vi "FetchImageSet (SubVI).vi"(8 "error in (no error)":errorcluster, 10 "Naming Convention":string="*.png", 11 "Images Directory":path=path "E:/XYZstage+Camera_CollectedImages/12-16-2016/noStaveMount/toolingpins_images") -> (0 "error out":errorcluster, 2 "Image Array":T1[](array[typedef]), 3 "Filenames Array":string[](array[string]))   [LabVIEW 2016]
uses:
  <vilib>/vision/Image Controls.llb/IMAQ Image.ctl
  <vilib>/regexp/Match Regular Expression.xnode
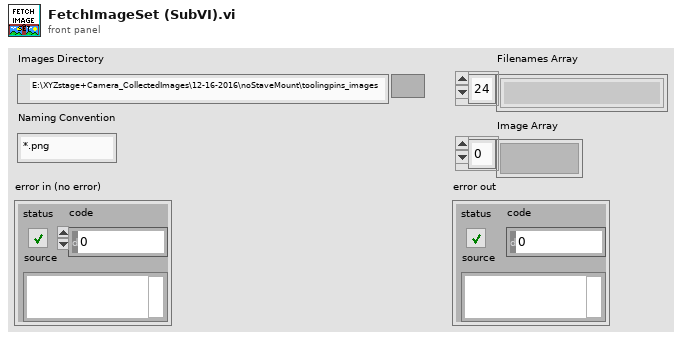
[diagram p1: front panel]
types:
  T1 = typedef "IMAQ Image.ctl" = refnum<image>
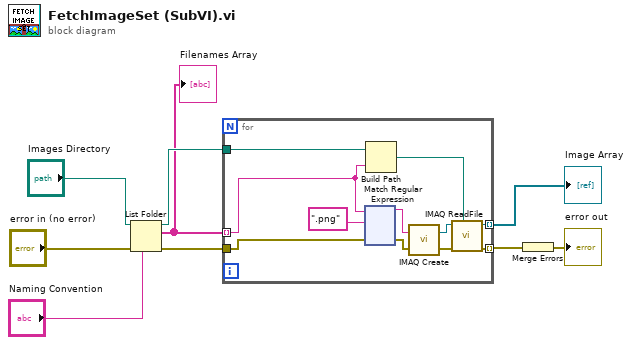
[diagram p0: block diagram]
diagram:
  n1 = List Folder(path="Images Directory", pattern="Naming Convention", error in="error in (no error)") -> (path out=w5:path, filenames=w1:string[], error out=w6:errorcluster)  [unwired: 1 in, 1 out]
  "Filenames Array" <- w1
  n2 = for {
    tunnel: w1 -> [w14] mode=indexing
    tunnel: w5 -> [w20]
    tunnel: w6 -> [w11]
    tunnel: [w16] -> w8 mode=indexing
    tunnel: [w15] -> w7 mode=indexing
    n3 = xnode "Match Regular Expression"("input string"=w14, "regular expression"=".png", "error in"=w11) -> ("before match"=w12:string, "error out"=w10:errorcluster)  [unwired: 3 in, 3 out]
    n4 = Build Path(base path=w20, name or relative path=w14) -> (appended path=w17:path)
    n5 = call "IMAQ Create"("Image Name"=w12, "error in (no error)"=w10) -> ("New Image"=w18:T1, "error out"=w19:errorcluster)  [unwired: 3 in]
    n6 = call "IMAQ ReadFile"("File Path"=w17, "error in (no error)"=w19, "Image"=w18) -> ("error out"=w15:errorcluster, "Image Out"=w16:T1)  [unwired: 4 in, 3 out]
  }
  "Image Array" <- w8
  n7 = Merge Errors(w7) -> (→"error out":errorcluster)
